vi "Phaeron Process Template.vi"() -> ()   [LabVIEW 2013]
uses:
  <vilib>/NI/AMC/Read Next Message.vi
  <vilib>/NI/AMC/Create Single Message.vi
  <vilib>/NI/AMC/Update Message Routing Info.vi
  <vilib>/NI/AMC/Read Termination Message.vi
  <vilib>/NI/AMC/Globals.vi
  <vilib>/NI/AMC/Send Message.vi
  <vilib>/NI/AMC/AMC.lvlib
panel:
  in  "Initialized?":refnum<k4>
  out "error out":errorcluster
  in  "error in (no error)":errorcluster
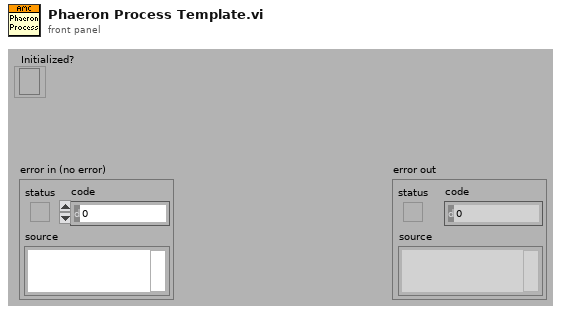
[diagram p1: front panel]
types:
  T1 = typedef "AMC.lvlib/Message Queue.ctl" = refnum<queue>
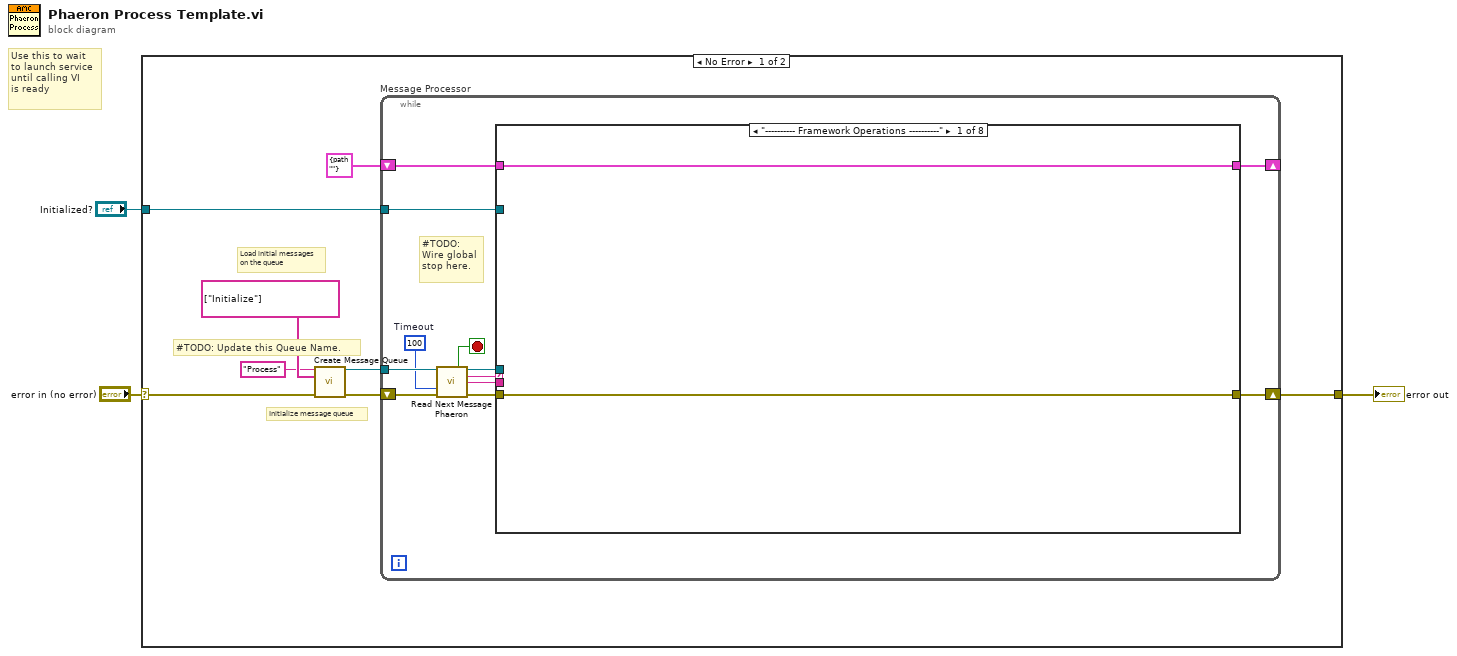
[diagram p0: block diagram]
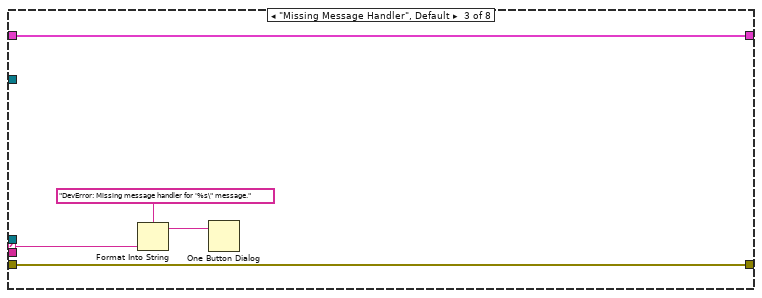
[diagram p3: hidden frame]
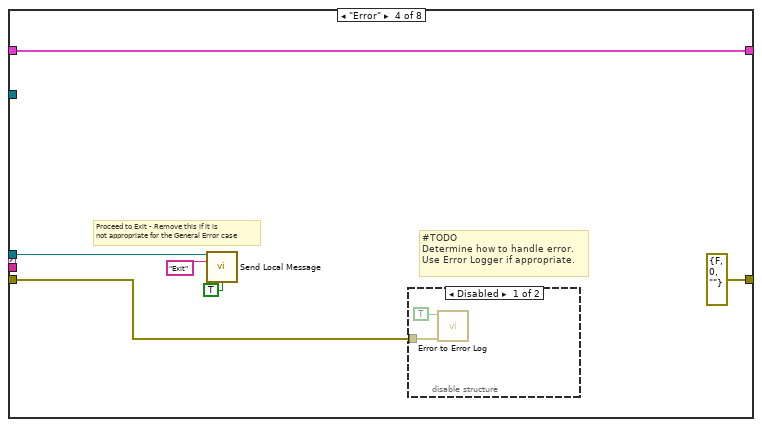
[diagram p4: hidden frame]
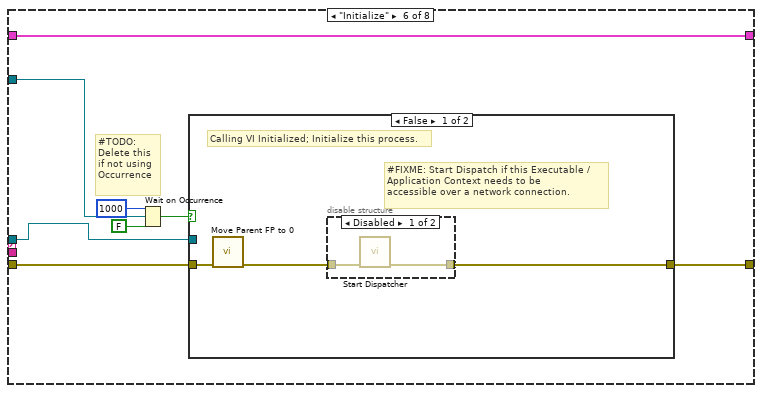
[diagram p7: hidden frame]
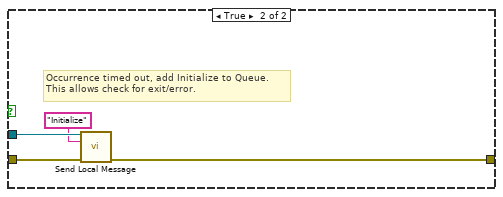
[diagram p9: hidden frame]
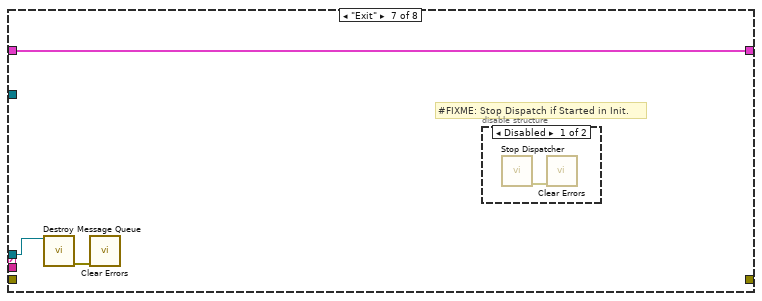
[diagram p10: hidden frame]
diagram:
  # "Use this to wait\nto launch service\nuntil calling VI\nis ready"
  n1 = case shown="No Error" "error in (no error)" {
    selector: "error in (no error)" -> [w6 w67]
    tunnel: [w5 w67] -> w2
    tunnel: "Initialized?" -> [w4 _]
    frame No Error {
      # "#TODO: Update this Queue Name."
      # "Initialize message queue"
      # "Load initial messages\non the queue"
      n2 = call <vilib>:"Create Message Queue.vi"("message queue name"="Process", "initial message names"=string[] ["Initialize"], "error in"=w6) -> ("message queue out"=w9:T1, "error out"=w10:errorcluster)  [unwired: 11 in]
      n3 = while "Message Processor" {
        shift-left: w10 -> [w17]
        shift-right: [w21] -> w5
        tunnel: w9 -> [w18]
        shift-left: cluster{"CurrentFile":path} {"CurrentFile"=path ""} ("State Variables") -> [w23]
        shift-right: [w22] -> _
        tunnel: w4 -> [w12]
        stop <- w20 stop-if-true
        w13 = 100  # Timeout
        # "#TODO:\nWire global\nstop here."
        n4 = call "Read Next Message Phaeron.vi"("message queue in"=w18, "timeout (1 ms)"=w13, "error in"=w17) -> ("exit process?"=w20:bool, "message queue out"=w19:T1, "message name"=w15:string, "message value"=w14:string, "error out"=w16:errorcluster)  [unwired: 5 in, 3 out]
        n5 = case shown="\"---------- Framework Operations ----------\"" w15 {
          selector: w15 -> [_ _ w30 _ _ _ _ _]
          tunnel: [w25 w27 w32 w38 w42 w50 w63 w66] -> w22
          tunnel: w23 -> [w25 w27 w32 w38 w42 w50 w63 w66]
          tunnel: w19 -> [_ _ _ w34 _ w44 w62 _]
          tunnel: w16 -> [w24 w26 w31 w33 w41 w43 _ w65]
          tunnel: [w24 w26 w31 errorcluster {"status"=FALSE, "code"=0, "source"=""} ("error out") w41 w46 _ w65] -> w21
          tunnel: w14 -> [_ _ _ _ _ _ _ _]
          tunnel: w12 -> [_ _ _ _ _ w45 _ _]
          frame "---------- Framework Operations ----------" {
          }
          frame "", "Idle" {
          }
          frame "Missing Message Handler", Default {
            n6 = Format Into String(format string="DevError: Missing message handler for '%s\" message." ("message"), w30) -> (resulting string=w28:string)  [unwired: 2 in, 1 out]
            n7 = One Button Dialog(message=w28) -> ()  [unwired: 2 out]
          }
          frame "Error" {
            # "#TODO\nDetermine how to handle error.\nUse Error Logger if appropriate."
            # "Proceed to Exit - Remove this if it is\nnot appropriate for the General Error case"
            n8 = call <vilib>:"Send Local Message.vi"("message queue in"=w34, "message name"="Exit", "priority message (F)"=TRUE) -> ()  [unwired: 10 in, 3 out]
            n9 = disable-structure shown="Disabled" {
              disable-tunnel: w33 -> [w40 _]
              frame Disabled {
                n10 = call "Error to Error Log.vi"("error in (no error)"=w40, "Clear?"=TRUE) -> ()  [unwired: 8 in, 2 out]
              }
              frame Enabled {
              }
            }
          }
          frame "---------- Generic Operations ----------" {
          }
          frame "Initialize" {
            # "#TODO:\nDelete this\nif not using\nOccurrence"
            n11 = Wait on Occurrence(1:FALSE ("ignore previous (T)"), 2:w45, 3:1000 ("ms timeout (-1)")) -> (0:w47:bool)
            n12 = case shown="False" w47 {
              tunnel: w43 -> [w53 w60]
              tunnel: [w51 w59] -> w46
              tunnel: w44 -> [_ w58]
              frame False {
                # "#FIXME: Start Dispatch if this Executable /\nApplication Context needs to be\naccessible over a network connection."
                # "Calling VI Initialized; Initialize this process."
                n13 = call "Move Parent FP to 0.vi"("error in"=w53) -> ("error out"=w52:errorcluster)  [unwired: 10 in]
                n14 = disable-structure shown="Disabled" {
                  disable-tunnel: w52 -> [w55 w56]
                  disable-tunnel: [w54 w56] -> w51
                  frame Disabled {
                    n15 = call <vilib>:"Start Dispatcher.vi"("error in"=w55) -> ("error out"=w54:errorcluster)  [unwired: 12 in, 2 out]
                  }
                  frame Enabled {
                  }
                }
              }
              frame True {
                # "Occurrence timed out, add Initialize to Queue.\nThis allows check for exit/error."
                n16 = call <vilib>:"Send Local Message.vi"("message queue in"=w58, "message name"="Initialize", "error in"=w60) -> ("error out"=w59:errorcluster)  [unwired: 10 in, 2 out]
              }
            }
          }
          frame "Exit" {
            # "#FIXME: Stop Dispatch if Started in Init."
            n17 = call <vilib>:"Destroy Message Queue.vi"("message queue in"=w62) -> ("error out"=w61:errorcluster)  [unwired: 12 in, 2 out]
            n18 = call <vilib>:"Clear Errors.vi"("error in (no error)"=w61) -> ()  [unwired: 6 in, 1 out]
            n19 = disable-structure shown="Disabled" {
              frame Disabled {
                n20 = call <vilib>:"Stop Dispatcher.vi"() -> ("error out"=w64:errorcluster)  [unwired: 15 in]
                n21 = call <vilib>:"Clear Errors.vi"("error in (no error)"=w64) -> ()  [unwired: 6 in, 1 out]
              }
              frame Enabled {
              }
            }
          }
          frame "---------- Application Operations ----------" {
          }
        }
      }
    }
    frame Error {
    }
  }
  "error out" <- w2
